vi "New.vi"(5 "ExpandSize (starting size)":i32=-1, 7 "CollapseDirection":T1, 8 "error in (no error)":errorcluster, 10 "Pane":refnum<vi>, 11 "Splitter":refnum<vi>) -> (0 "error out":errorcluster, 3 "CollapsePanel out":refnum<class "CollapsePanel.lvclass">)   [LabVIEW 2021, in "CollapsePanel.lvclass"]
uses:
  CollapsePanel.lvclass
  collapse direction.ctl
  CollapsePanel.lvclass/CollapsePanel.ctl
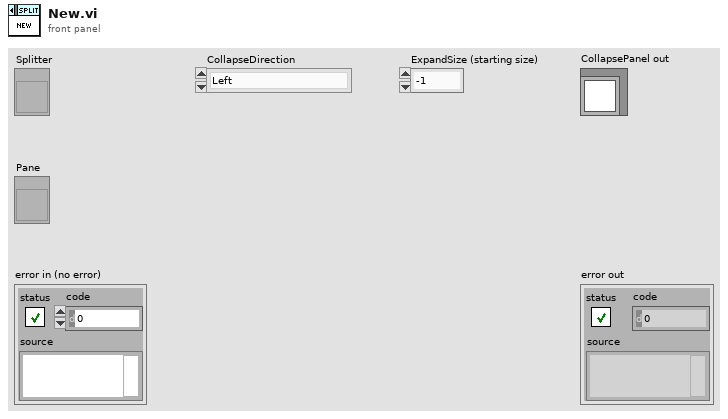
[diagram p1: front panel]
types:
  T1 = typedef "CollapsePanel.lvclass/collapse direction.ctl" = enum16{"Left", "Right", "Up", "Down"}
  T2 = enum16{"No Scaling", "Scale All Objects", "Scale Single Object"}
  T3 = typedef "LVBoundsTypeDef.ctl" = cluster{"Width":u32, "Height":u32}
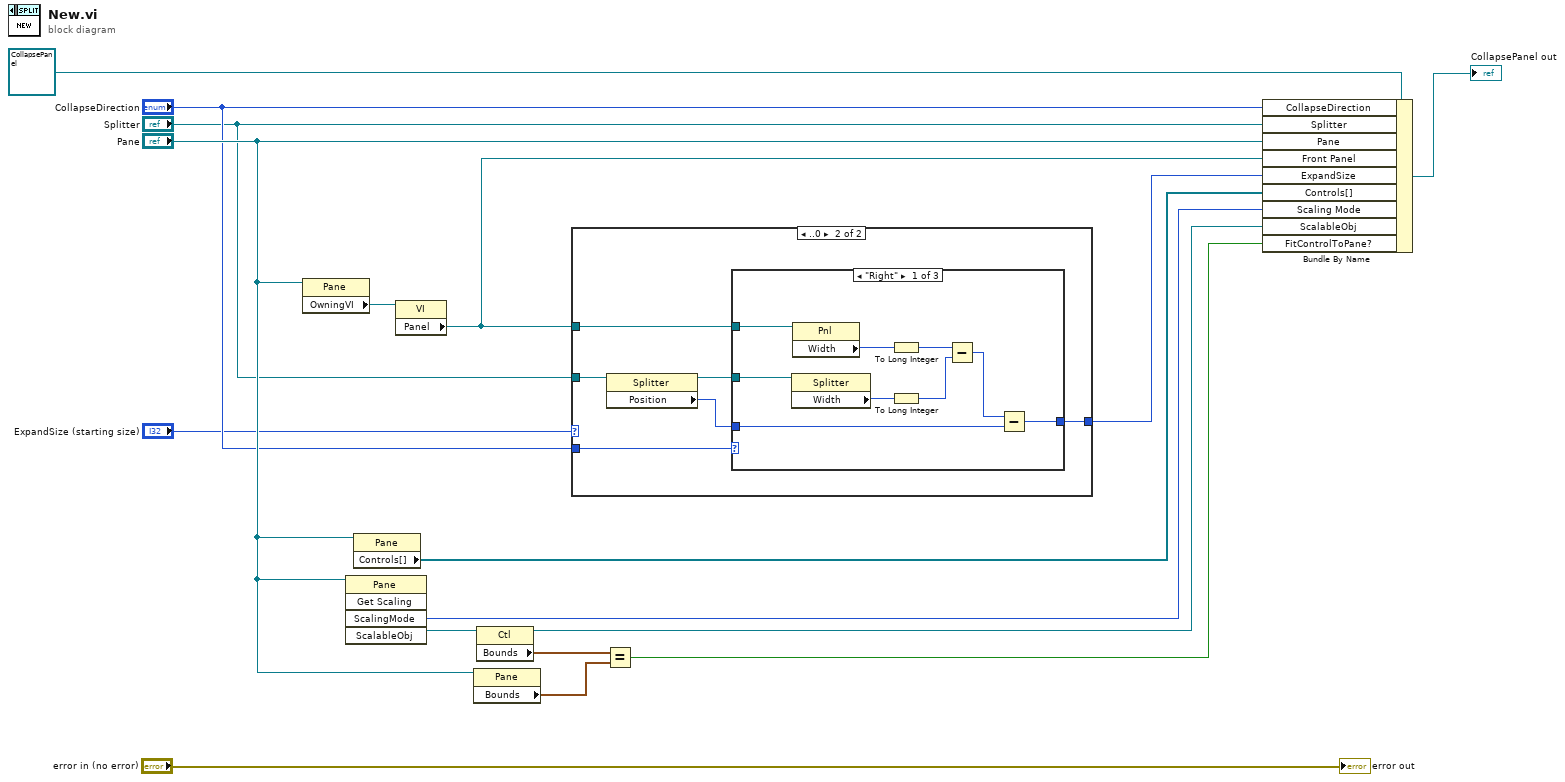
[diagram p0: block diagram]
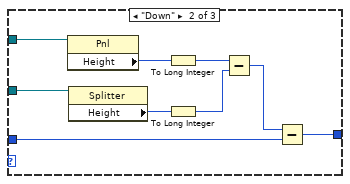
[diagram p3: hidden frame]
diagram:
  n1 = property class="Pane"(reference="Pane") -> ("OwningVI"=w15:refnum<vi>)  [unwired: 1 in, 2 out]
  n2 = invoke class="Pane" method="Get Scaling"(reference="Pane") -> ("ScalingMode"=w7:T2, "ScalableObj"=w13:refnum<vi>)  [unwired: 4 in, 3 out]
  n3 = property class="Pane"(reference="Pane") -> ("Controls[]"=w9:refnum<vi>[])  [unwired: 1 in, 2 out]
  n4 = property class="VI"(reference=w15) -> ("Panel"=w5:refnum<vi>)  [unwired: 1 in, 2 out]
  n5 = property class="Pane"(reference="Pane") -> ("Bounds"=w11:T3)  [unwired: 1 in, 2 out]
  n6 = property class="Ctl"(reference=w13) -> (reference out=w6:refnum<vi>, "Bounds"=w12:T3)  [unwired: 1 in, 1 out]
  n7 = case shown="..0" "ExpandSize (starting size)" {
    selector: "ExpandSize (starting size)" -> [w18 _]
    tunnel: w5 -> [_ w24]
    tunnel: "CollapseDirection" -> [_ w21]
    tunnel: "Splitter" -> [_ w20]
    tunnel: [w18 w19] -> w2
    frame Default {
    }
    frame ..0 {
      n8 = property class="Splitter"(reference=w20) -> (reference out=w23:refnum<vi>, "Position"=w22:i32)  [unwired: 1 in, 1 out]
      n9 = case shown="\"Right\"" w21 {
        tunnel: w24 -> [w33 w42 _]
        tunnel: w23 -> [w32 w41 _]
        tunnel: [w25 w34 w43] -> w19
        tunnel: w22 -> [w26 w35 w43]
        frame "Right" {
          n10 = property class="Splitter"(reference=w32) -> ("Width"=w30:u32)  [unwired: 1 in, 2 out]
          n11 = property class="Pnl"(reference=w33) -> ("Width"=w31:u32)  [unwired: 1 in, 2 out]
          n12 = To Long Integer(number=w31) -> (32bit integer=w28:i32)
          n13 = To Long Integer(number=w30) -> (32bit integer=w29:i32)
          n14 = Subtract(x=w28, y=w29) -> (x-y=w27:i32)
          n15 = Subtract(x=w27, y=w26) -> (x-y=w25:i32)
        }
        frame "Down" {
          n16 = property class="Pnl"(reference=w42) -> ("Height"=w40:u32)  [unwired: 1 in, 2 out]
          n17 = property class="Splitter"(reference=w41) -> ("Height"=w39:u32)  [unwired: 1 in, 2 out]
          n18 = To Long Integer(number=w40) -> (32bit integer=w37:i32)
          n19 = To Long Integer(number=w39) -> (32bit integer=w38:i32)
          n20 = Subtract(x=w37, y=w38) -> (x-y=w36:i32)
          n21 = Subtract(x=w36, y=w35) -> (x-y=w34:i32)
        }
        frame "Left", "Up" {
        }
      }
    }
  }
  n22 = Equal?(x=w12, y=w11) -> (x = y?=w8:bool)
  n23 = Bundle By Name(cluster=refnum<class "CollapsePanel.lvclass"> refnum ("CollapsePanel out"), "CollapseDirection"="CollapseDirection", "Splitter"="Splitter", "Pane"="Pane", "Front Panel"=w5, "ExpandSize"=w2, "Controls[]"=w9, "Scaling Mode"=w7, "ScalableObj"=w6, "FitControlToPane?"=w8) -> (→"CollapsePanel out":refnum<class "CollapsePanel.lvclass">)
  "error out" <- "error in (no error)"
